vi "subConvertLabVIEWBasedPath.vi"(10 "Parent":path, 11 "Path in":path) -> (3 "Path":path)   [LabVIEW 2020, in "CommonHelpers.lvlib"]
uses:
  CommonHelpers.lvlib
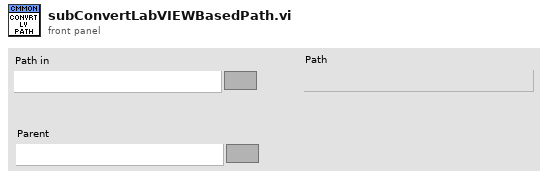
[diagram p1: front panel]
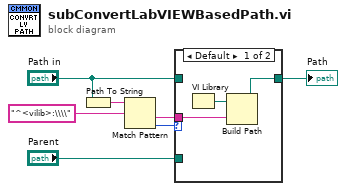
[diagram p0: block diagram]
diagram:
  n1 = Path To String(path="Path in") -> (string=w7:string)
  n2 = Match Pattern(string=w7, regular expression="^<vilib>:\\\\") -> (after substring=w2:string, offset past match=w5:i32)  [unwired: 1 in, 2 out]
  n3 = case shown="Default" w5 {
    tunnel: [w8 w11] -> w4
    tunnel: "Path in" -> [_ w11]
    tunnel: w2 -> [w9 _]
    tunnel: "Parent" -> [_ _]
    frame Default {
      n4 = VI Library() -> (path=w10:path)
      n5 = Build Path(base path=w10, name or relative path=w9) -> (appended path=w8:path)
    }
    frame -1 {
    }
  }
  "Path" <- w4
